vi "niDTS BT INSTR TX UTIL Convert Burst sync.vi"(7 "Burst Sync":T1(ring)=enum."PREamble") -> (8 "BurstSyncType":enum16{"PREamble", "NONE"}(ring))   [LabVIEW 2015, in "niDTS BT.lvlib" / "niDTS BT INSTR TX.lvclass"]
uses:
  niDTS BT INSTR TX.lvclass
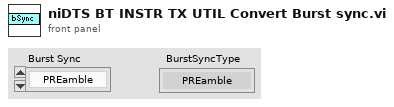
[diagram p1: front panel]
types:
  T1 = enum16{"ACODe", "RFAMplitude", "NONE", "PREamble", "AADRess"}
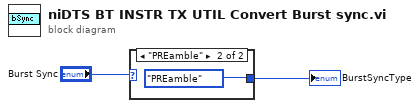
[diagram p0: block diagram]
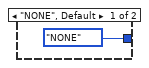
[diagram p2: hidden frame]
diagram:
  n1 = case shown="\"PREamble\"" "Burst Sync" {
    tunnel: [enum16{"PREamble", "NONE"}."NONE" ("CONFigure:RFSA:BLUetooth:BurstSyncType") enum16{"PREamble", "NONE"}."PREamble" ("CONFigure:RFSA:BLUetooth:BurstSyncType")] -> w1
    frame "NONE", Default {
    }
    frame "PREamble" {
    }
  }
  "BurstSyncType" <- w1
